vi "CC Get All Files for Image.vi"(8 "error in (no error)":errorcluster, 11 "path":path) -> (0 "error out":errorcluster, 3 "Files for image":path[](array[path]))   [LabVIEW 2024]
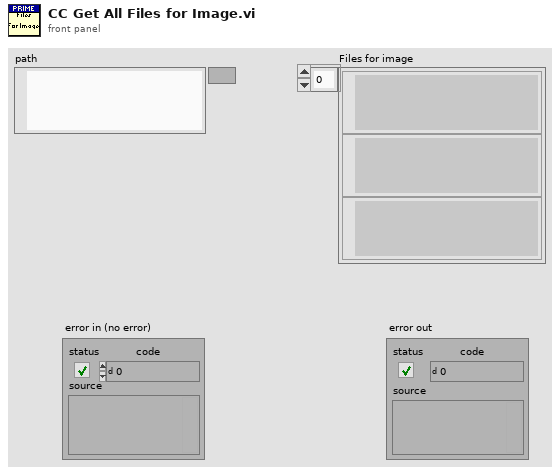
[diagram p1: front panel]
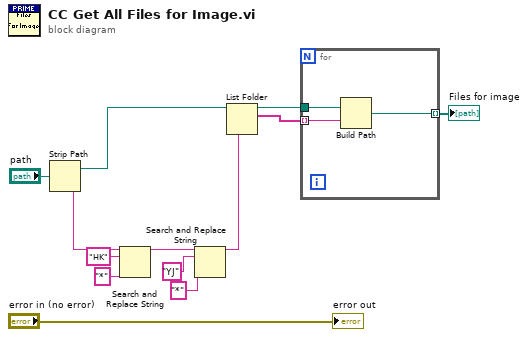
[diagram p0: block diagram]
diagram:
  n1 = Strip Path(path="path") -> (stripped path=w12:path, name=w7:string)
  n2 = Search and Replace String(input string=w7, search string="HK", replace string="*" ("replace string (\"\")")) -> (result string=w2:string)  [unwired: 5 in, 3 out]
  n3 = Search and Replace String(input string=w2, search string="YJ", replace string="*" ("replace string (\"\")")) -> (result string=w1:string)  [unwired: 5 in, 3 out]
  n4 = List Folder(path=w12, pattern=w1) -> (path out=w10:path, filenames=w9:string[])  [unwired: 2 in, 2 out]
  n5 = for {
    tunnel: w10 -> [w16]
    tunnel: w9 -> [w15] mode=indexing
    tunnel: [w14] -> w8 mode=indexing
    n6 = Build Path(base path=w16, name or relative path=w15) -> (appended path=w14:path)
  }
  "Files for image" <- w8
  "error out" <- "error in (no error)"
